vi "Teleop.vi"(8 "error in":errorcluster, 10 "Match Info":T1={"Autonomous Elapsed Seconds"=0.0, "TeleOp Elapsed Seconds"=0.0, "Disabled Elapsed Seconds"=0.0, "Visited Autonomous"=FALSE, "Visited TeleOp"=FALSE, "Visited Disabled"=FALSE, "Autonomous Settings"={"Autonomous Style"=enum."Independent", "VI Refnum"=refnum}}, 11 "Call Context":T2) -> (0 "error out":errorcluster)   [LabVIEW 2013]
doc: "This VI is called for each TeleOp packet received from the DS where the robot is not disabled. It is often used to read from the joysticks and update I/O or to update setpoints for timed control loops. It should complete and return within 20 milliseconds or it may miss DS packets."
uses:
  <vilib>/Rock Robotics/WPI/DriverStation/WPI_DriverStationDerivedRobotMode.ctl
  <vilib>/Rock Robotics/WPI/DriverStation/WPI_DriverStationMatch Info.ctl
  <vilib>/Rock Robotics/WPI/Relay/WPI_RelayValue.ctl
  Robot Global Data.vi
  <vilib>/Rock Robotics/WPI/Joystick/WPI_JoystickGetSetRefNum.vi
  <vilib>/Rock Robotics/WPI/RobotDrive/WPI_RobotDriveArcadeDrive_Standard(NoSaturation).vi
  <vilib>/Rock Robotics/WPI/RobotDrive/WPI_RobotDriveGetSetRefNum.vi
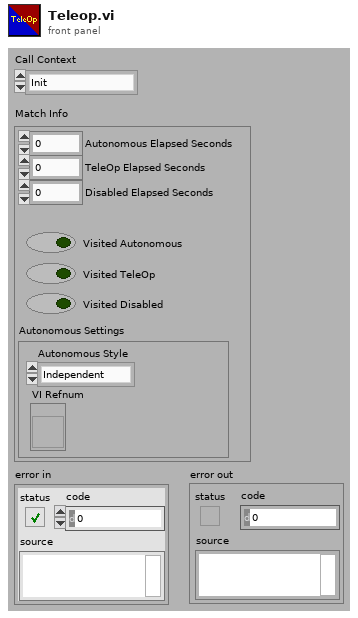
[diagram p1: front panel]
types:
  T1 = typedef "WPI_DriverStationMatch Info.ctl" = cluster{"Autonomous Elapsed Seconds":dbl, "TeleOp Elapsed Seconds":dbl, "Disabled Elapsed Seconds":dbl, "Visited Autonomous":bool, "Visited TeleOp":bool, "Visited Disabled":bool, "Autonomous Settings":cluster{"Autonomous Style":enum16{"Iterative", "Independent"}, "VI Refnum":refnum<vi>}}
  T2 = typedef "WPI_DriverStationDerivedRobotMode.ctl" = enum16{"Init", "Execute", "Stop"}
  T3 = typedef "WPI_RelayValue.ctl" = enum16{"Off", "On", "Forward", "Reverse"}
  T4 = typedef "WPI_JoystickDevRef.ctl" = cluster{"Device":T5}
  T5 = typedef "WPI_JoystickDeviceEnum.ctl" = enum16{"USB 1", "USB 2", "USB 3", "USB 4", "Kinect 1", "Kinect 2"}
  T6 = typedef "WPI_JoystickButtonState.ctl" = cluster{"Button 1":bool, "Button 2":bool, "Button 3":bool, "Button 4":bool, "Button 5":bool, "Button 6":bool, "Button 7":bool, "Button 8":bool, "Button 9":bool, "Button 10":bool, "Button 11":bool, "Button 12":bool}
  T7 = cluster{"axis 1 (x)":dbl, "axis 2 (y)":dbl, "axis 3 (throttle)":dbl, "axis 4":dbl, "axis 5":dbl, "axis 6":dbl}
  T8 = typedef "WPI_RobotDriveDevRef.ctl" = cluster{"DevStatus":errorcluster, "Motors[]":T9[], "Square Inputs":bool, "Max Output":dbl, "Isochronous":bool}
  T9 = typedef "WPI_MotorControlDeviceRef.ctl" = cluster{"DeviceStatus":errorcluster, "Type":enum16{"PWM", "CAN"}, "PWM":cluster{"Digital Module":T10, "PWM Channel":T11, "DeadBand":T12}, "CAN":cluster{"Device Number":u8, "Control Mode":T13, "Semaphore":T14, "Max Vout":dbl}, "Invert":bool, "TransformRef":T15, "InvTransformRef":T15}
  T10 = typedef "FPGA_TypedefDigitalModule.ctl" = enum16{"Digital Module 1", "Digital Module 2"}
  T11 = typedef "FPGA_DIOPWMChannel.ctl" = enum8{"PWM 1", "PWM 2", "PWM 3", "PWM 4", "PWM 5", "PWM 6", "PWM 7", "PWM 8", "PWM 9", "PWM 10", "Invalid"}
  T12 = typedef "WPI_PWMDeadband.ctl" = cluster{"Name":string, "maxPositivePwm":i32, "minPositivePwm":i32, "centerPwm":i32, "maxNegativePwm":i32, "minNegativePwm":i32, "angularRange":u16}
  T13 = typedef "WPI_CANJaguar_ControlMode.ctl" = enum8{"Percent VBus", "Current", "Speed", "Position", "Voltage"}
  T14 = typedef "Semaphore RefNum" = refnum<k1>
  T15 = typedef "WPI_PWMTransform_ConPane.ctl" = refnum<vi>
  T16 = typedef "WPI_ServoDeviceRef.ctl" = cluster{"DeviceStatus":errorcluster, "Digital Module":T10, "PWM Channel":T11, "DeadBand":T12}
  T17 = typedef "WPI_RelayDevRef.ctl" = cluster{"DevStatus":errorcluster, "Relay Channel":T18, "Digital Module":T10, "Relay Direction":T19}
  T18 = typedef "FPGA_DIORelayChannel.ctl" = enum8{"Relay 1", "Relay 2", "Relay 3", "Relay 4", "Relay 5", "Relay 6", "Relay 7", "Relay 8", "Invalid"}
  T19 = typedef "WPI_RelayDirection.ctl" = enum16{"Both directions", "Forward only", "Reverse only"}
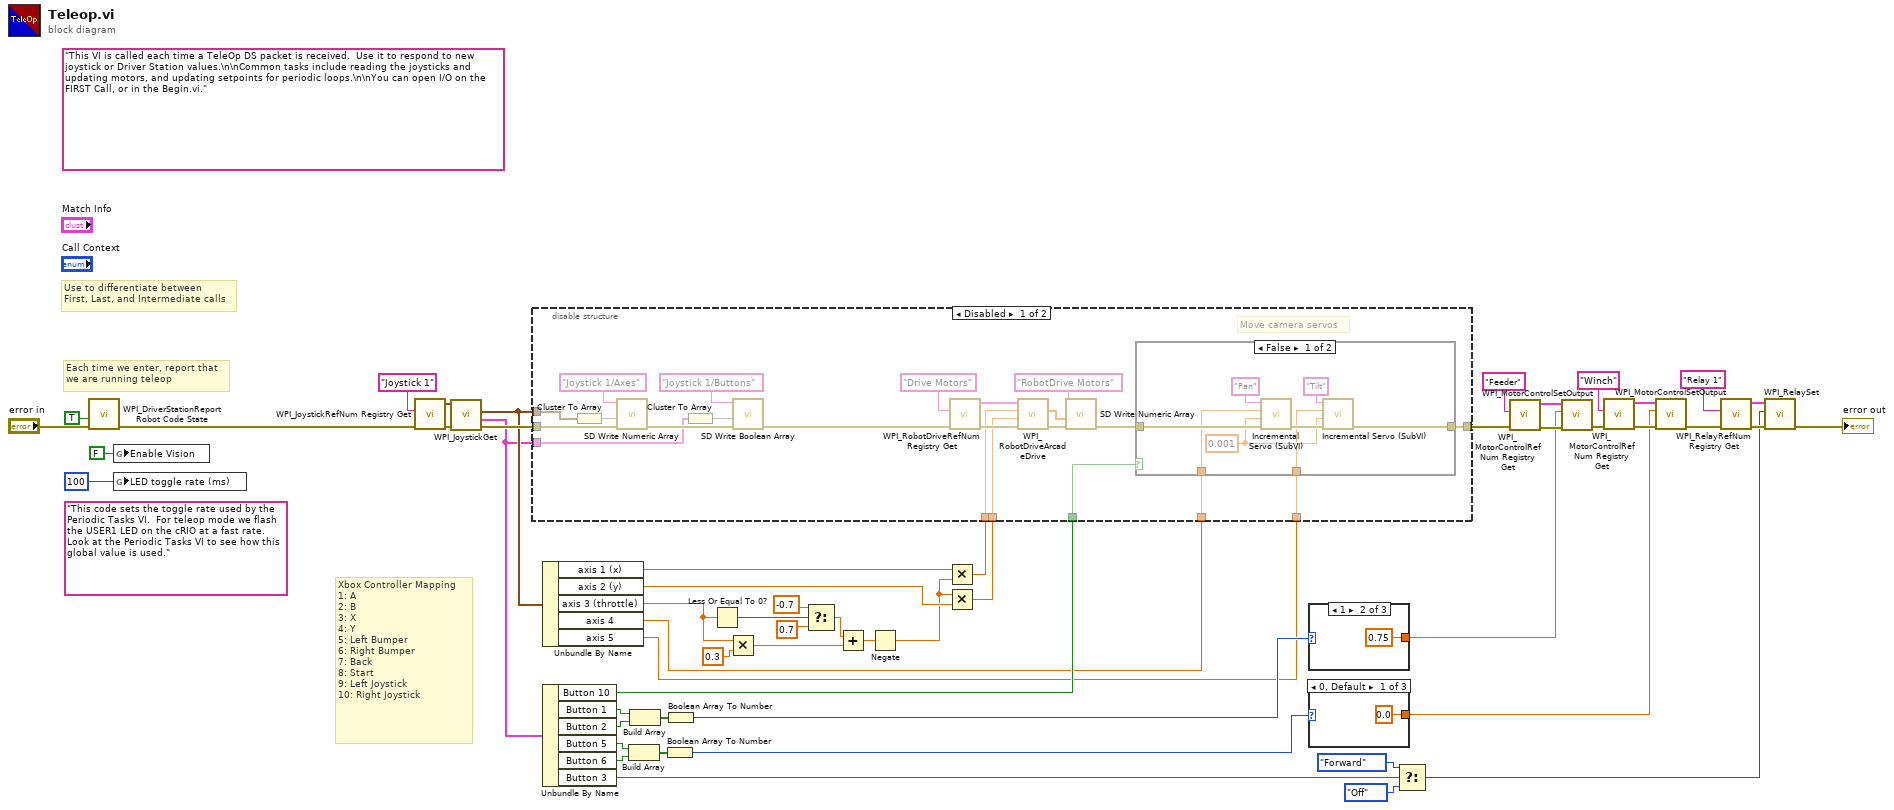
[diagram p0: block diagram]
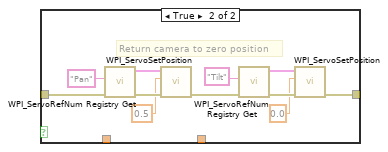
[diagram p2: hidden frame]
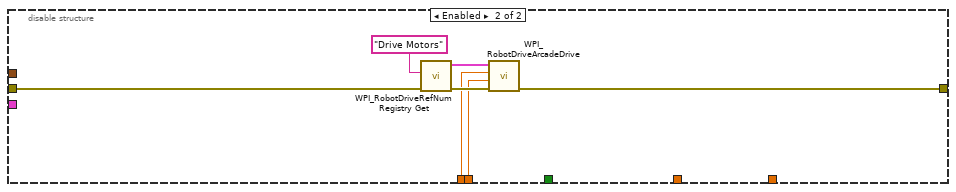
[diagram p3: hidden frame]
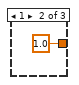
[diagram p4: hidden frame]
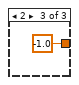
[diagram p5: hidden frame]
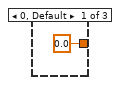
[diagram p6: hidden frame]
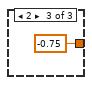
[diagram p7: hidden frame]
diagram:
  (unwired) "This code sets the toggle rate used by the Periodic Tasks VI.  For teleop mode we flash the USER1 LED on the cRIO at a fast rate.  Look at the Periodic Tasks VI to see how this global value is used."
  (unwired) "This VI is called each time a TeleOp DS packet is received.  Use it to respond to new joystick or Driver Station values.\n\nCommon tasks include reading the joysticks and updating motors, and updating setpoints for periodic loops.\n\nYou can open I/O on the FIRST Call, or in the Begin.vi."
  # "Xbox Controller Mapping\n1: A\n2: B\n3: X\n4: Y\n5: Left Bumper\n6: Right Bumper\n7: Back\n8: Start\n9: Left Joystick\n10: Right Joystick"
  # "Each time we enter, report that\nwe are running teleop"
  # "Use to differentiate between\nFirst, Last, and Intermediate calls"
  n1 = call <vilib>:"WPI_DriverStationReport Robot Code State.vi"("error in (no error)"="error in", "TeleOp"=TRUE ("Autonomous")) -> ("error out"=w29:errorcluster)  [unwired: 9 in]
  n2 = global write "Robot Global Data.vi" "Enable Vision"(FALSE ("Enable Vision")) -> ()
  n3 = global write "Robot Global Data.vi" "LED toggle rate (ms)"(u32 100 ("LED ms toggle rate")) -> ()
  n4 = call <vilib>:"WPI_JoystickRefNum Registry Get.vi"("error in (no error)"=w29, "refnum name"="Joystick 1") -> ("error out"=w11:errorcluster, "JoystickDevRef"=w10:T4)  [unwired: 8 out]
  n5 = call <vilib>:"WPI_JoystickGet.vi"("JoystickDevRef"=w10) -> ("Buttons"=w8:T6, "Axes"=w9:T7)  [unwired: 1 in, 4 out]
  n6 = Unbundle By Name(w9) -> ("axis 1 (x)"=w50:dbl, "axis 2 (y)"=w49:dbl, "axis 3 (throttle)"=w45:dbl, "axis 4"=w37:dbl, "axis 5"=w36:dbl)
  n7 = Unbundle By Name(w8) -> ("Button 10"=w39:bool, "Button 1"=w43:bool, "Button 2"=w42:bool, "Button 5"=w33:bool, "Button 6"=w34:bool, "Button 3"=w31:bool)
  n8 = Build Array(w33, w34) -> (w35:bool[])
  n9 = Build Array(w43, w42) -> (w41:bool[])
  n10 = Boolean Array To Number(Boolean array=w35) -> (number=w32:u32)
  n11 = Boolean Array To Number(Boolean array=w41) -> (number=w38:u32)
  n12 = Less Or Equal To 0?(x=w45) -> (x <= 0?=w6:bool)
  n13 = Multiply(x=w45, y=0.3) -> (x*y=w7:dbl)
  n14 = Select(t=-0.7, s=w6, f=0.7) -> (s? t:f=w3:dbl)
  n15 = Add(x=w3, y=w7) -> (x+y=w2:dbl)
  n16 = Negate(x=w2) -> (-x=w1:dbl)
  n17 = Multiply(x=w50, y=w1) -> (x*y=w47:dbl)
  n18 = Multiply(x=w1, y=w49) -> (x*y=w46:dbl)
  n19 = disable-structure shown="Disabled" {
    disable-tunnel: w11 -> [w69 w96]
    disable-tunnel: w47 -> [w65 w98]
    disable-tunnel: w46 -> [w64 w97]
    disable-tunnel: w39 -> [w61 _]
    disable-tunnel: w37 -> [w59 _]
    disable-tunnel: w36 -> [w58 _]
    disable-tunnel: [w56 w95] -> w25
    disable-tunnel: w9 -> [w55 _]
    disable-tunnel: w8 -> [w54 _]
    frame Disabled {
      # "Move camera servos"
      n20 = Cluster To Array(cluster=w55) -> (array=w73:dbl[])
      n21 = call <vilib>:"SD Write Numeric Array.vi"("error in"=w69, "Numeric Array"=w73, "Name"="Joystick 1/Axes") -> ("error out"=w71:errorcluster)  [unwired: 7 in, 1 out]
      n22 = Cluster To Array(cluster=w54) -> (array=w70:bool[])
      n23 = call <vilib>:"SD Write Boolean Array.vi"("error in"=w71, "Boolean Array"=w70, "Name"="Joystick 1/Buttons") -> ("error out"=w60:errorcluster)  [unwired: 7 in, 1 out]
      n24 = call <vilib>:"WPI_RobotDriveRefNum Registry Get.vi"("error in (no error)"=w60, "refnum name"="Drive Motors") -> ("error out"=w68:errorcluster, "RobotDriveDevRef"=w67:T8)  [unwired: 8 out]
      n25 = call-poly <vilib>:"WPI_RobotDriveArcadeDrive.vi"("error in (no error)"=w68, "Y axis value"=w64, "X axis value"=w65, "RobotDriveDevRef"=w67) -> ("error out"=w66:errorcluster, "Motor Values"=w63:dbl[])  [unwired: 5 in, 1 out]
      n26 = call <vilib>:"SD Write Numeric Array.vi"("error in"=w66, "Numeric Array"=w63, "Name"="RobotDrive Motors") -> ("error out"=w62:errorcluster)  [unwired: 7 in, 1 out]
      n27 = case shown="False" w61 {
        tunnel: [w80 w85] -> w56
        tunnel: w62 -> [w79 w84]
        tunnel: w59 -> [w77 _]
        tunnel: w58 -> [w76 _]
        frame False {
          w78 = 0.001 ("Threshold")
          n28 = call "Incremental Servo (SubVI).vi"("error in (no error)"=w79, "Threshold"=w78, "Axis Value"=w77, "Servo refnum"="Pan") -> ("error out"=w83:errorcluster)  [unwired: 5 in]
          n29 = call "Incremental Servo (SubVI).vi"("error in (no error)"=w83, "Threshold"=w78, "Axis Value"=w76, "Servo refnum"="Tilt") -> ("error out"=w80:errorcluster)  [unwired: 5 in]
        }
        frame True {
          # "Return camera to zero position"
          n30 = call <vilib>:"WPI_ServoRefNum Registry Get.vi"("error in (no error)"=w84, "refnum name"="Pan") -> ("error out"=w93:errorcluster, "ServoDeviceRef"=w92:T16)  [unwired: 8 in]
          n31 = call <vilib>:"WPI_ServoSetPosition.vi"("error in (no error)"=w93, "Position"=0.5, "ServoDeviceRef"=w92) -> ("error out"=w87:errorcluster)  [unwired: 7 in, 1 out]
          n32 = call <vilib>:"WPI_ServoRefNum Registry Get.vi"("error in (no error)"=w87, "refnum name"="Tilt") -> ("error out"=w89:errorcluster, "ServoDeviceRef"=w90:T16)  [unwired: 8 in]
          n33 = call <vilib>:"WPI_ServoSetPosition.vi"("error in (no error)"=w89, "Position"=0.0, "ServoDeviceRef"=w90) -> ("error out"=w85:errorcluster)  [unwired: 7 in, 1 out]
        }
      }
    }
    frame Enabled {
      n34 = call <vilib>:"WPI_RobotDriveRefNum Registry Get.vi"("error in (no error)"=w96, "refnum name"="Drive Motors") -> ("error out"=w100:errorcluster, "RobotDriveDevRef"=w99:T8)  [unwired: 8 out]
      n35 = call-poly <vilib>:"WPI_RobotDriveArcadeDrive.vi"("error in (no error)"=w100, "Y axis value"=w97, "X axis value"=w98, "RobotDriveDevRef"=w99) -> ("error out"=w95:errorcluster)  [unwired: 5 in, 2 out]
    }
  }
  n36 = case shown="1" w38 {
    tunnel: [0.0 ("Output") 0.75 ("Output") -0.75 ("Output")] -> w24
    frame 0, Default {
    }
    frame 1 {
    }
    frame 2 {
    }
  }
  n37 = case shown="0, Default" w32 {
    tunnel: [0.0 ("Output") 1.0 ("Output") -1.0 ("Output")] -> w19
    frame 0, Default {
    }
    frame 1 {
    }
    frame 2 {
    }
  }
  n38 = Select(t=WPI_RelayValue."Forward" ("RelayValue"), s=w31, f=WPI_RelayValue."Off" ("RelayValue")) -> (s? t:f=w12:T3)
  n39 = call <vilib>:"WPI_MotorControlRefNum Registry Get.vi"("error in (no error)"=w25, "refnum name"="Feeder") -> ("error out"=w26:errorcluster, "MotorControlDevRef"=w27:T9)  [unwired: 8 in]
  n40 = call <vilib>:"WPI_MotorControlSetOutput.vi"("error in (no error)"=w26, "Output"=w24, "MotorControlDevRef"=w27) -> ("error out"=w21:errorcluster)  [unwired: 6 in, 2 out]
  n41 = call <vilib>:"WPI_MotorControlRefNum Registry Get.vi"("error in (no error)"=w21, "refnum name"="Winch") -> ("error out"=w20:errorcluster, "MotorControlDevRef"=w23:T9)  [unwired: 8 in]
  n42 = call <vilib>:"WPI_MotorControlSetOutput.vi"("error in (no error)"=w20, "Output"=w19, "MotorControlDevRef"=w23) -> ("error out"=w18:errorcluster)  [unwired: 6 in, 2 out]
  n43 = call <vilib>:"WPI_RelayRefNum Registry Get.vi"("error in (no error)"=w18, "refnum name"="Relay 1") -> ("error out"=w17:errorcluster, "RelayDevRef"=w16:T17)  [unwired: 8 in]
  n44 = call <vilib>:"WPI_RelaySet.vi"("error in (no error)"=w17, "RelayValue"=w12, "RelayDevRef"=w16) -> ("error out"=→"error out":errorcluster)  [unwired: 7 in, 1 out]
